vi "VCI_Transmit.vi"(7 "Buffer":T1[](array[typedef]), 8 "error in (no error)":errorcluster caption="错误输入（无错误）", 9 "CANIndex":u32, 10 "DevIndex":u32, 11 "DevType":T2=2 items=["USB-CAN"=2, "USB-CAN2"=3]) -> (0 "error out":errorcluster caption="错误输出", 3 "Return Val":T3=1 items=["OK"=1, "ERROR1"=0, "ERROR2"=-1])   [LabVIEW 2018, in "ControlCan.lvlib"]
uses:
  ControlCan.lvlib
  Return Val.ctl
  DevType.ctl
  VCI_CAN_OBJ.ctl
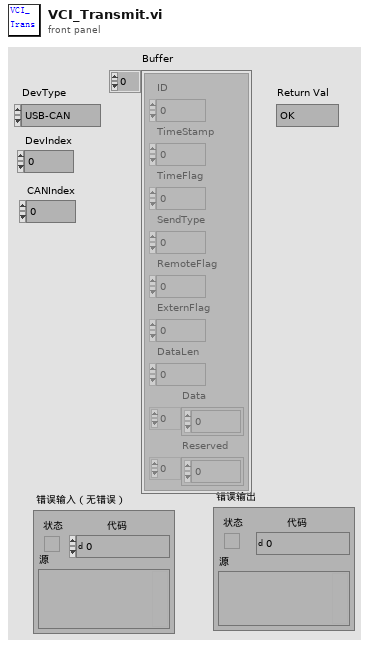
[diagram p1: front panel]
types:
  T1 = typedef "ControlCAN.lvlib/VCI_CAN_OBJ.ctl" = cluster{"ID":u32, "TimeStamp":u32, "TimeFlag":u8, "SendType":u8, "RemoteFlag":u8, "ExternFlag":u8, "DataLen":u8, "Data":u8[], "Reserved":u8[]}
  T2 = typedef "ControlCAN.lvlib/DevType.ctl" = u32
  T3 = typedef "ControlCAN.lvlib/Return Val.ctl" = i32
  T4 = typedef "ControlCAN.lvlib/VCI_CAN_OBJ_1.ctl" = cluster{"ID":u32, "TimeStamp":u32, "TimeFlag":u8, "SendType":u8, "RemoteFlag":u8, "ExternFlag":u8, "DataLen":u8, "Data 0":u8, "Data 1":u8, "Data 2":u8, "Data 3":u8, "Data 4":u8, "Data 5":u8, "Data 6":u8, "Data 7":u8, "Reserved 0":u8, "Reserved 1":u8, "Reserved 2":u8}
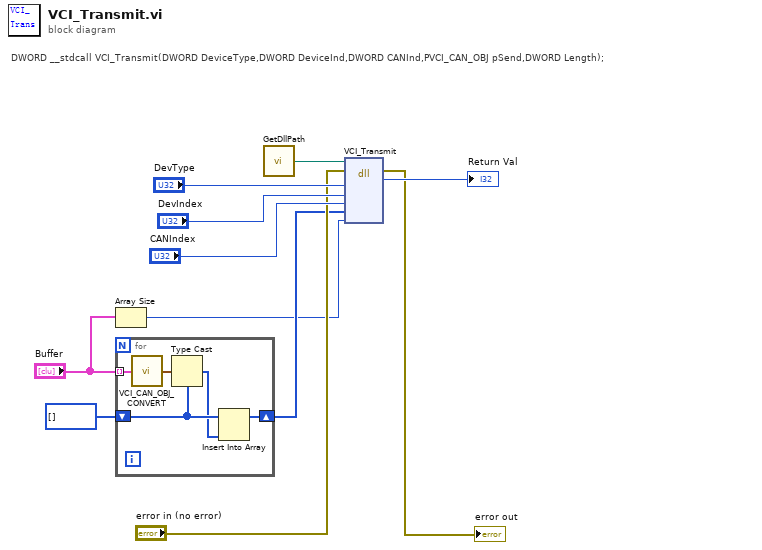
[diagram p0: block diagram]
diagram:
  # "DWORD __stdcall VCI_Transmit(DWORD DeviceType,DWORD DeviceInd,DWORD CANInd,PVCI_CAN_OBJ pSend,DWORD Length);"
  n1 = Array Size(array="Buffer") -> (size(s)=w2:i32)
  n2 = for {
    tunnel: "Buffer" -> [w16] mode=indexing
    shift-right: [w12] -> w3
    shift-left: u8[] [] ("pSend") -> [w14]
    n3 = call "VCI_CAN_OBJ_CONVERT.vi"("VCI_CAN_OBJ"=w16) -> ("VCI_CAN_OBJ_1"=w15:T4)
    n4 = Type Cast(type=w14, x=w15) -> (*(type *) &x=w13:u8[])
    n5 = Insert Into Array(array=w14, new element=w13) -> (w12:u8[])  [unwired: 1 in]
  }
  n6 = call "GetDllPath.vi"() -> ("DllPath"=w1:path)  [unwired: 1 out]
  n7 = dll-call lib="?" fn="VCI_Transmit"(path in=w1, error in="error in (no error)", "DevType"="DevType", "DevIndex"="DevIndex", "CANIndex"="CANIndex", "pSend"=w3, "Length"=w2) -> (error out=→"error out":errorcluster, "ReturnVal"=→"Return Val":i32)  [unwired: 6 in, 1 out]
